vi "探头测量值显示.vi"(11 "校准参数":u16(ring) caption="校准参数：" items=["pH", "DO", "浊度", "电导率", "叶绿素a", "藻密度", "ORP", "COD", "DO2", "氯化物", "氨氮", "水中油", "悬浮物"]) -> (0 "线性系数":cluster{bool, "K":sgl, "B":sgl}, 1 "信号值":sgl, 2 "检测值":sgl, 3 "序列号":string, 4 "检测值.格式字符串":string, 5 "温度补偿系数":cluster{bool, "温度补偿系数":sgl}, 6 "信号值.格式字符串":string, 7 "电极状态标志":u16)   [LabVIEW 2022 SP3, in "斯坦道多参数.lvlib"]
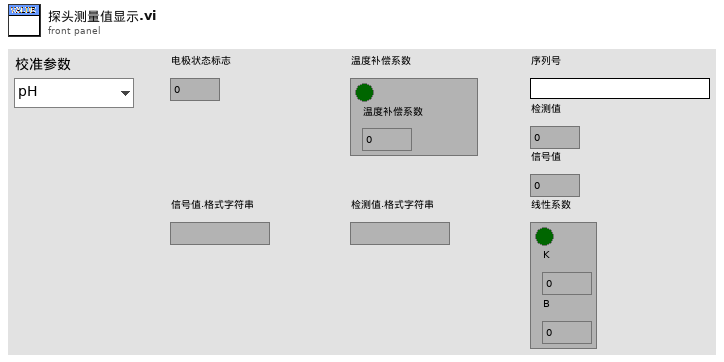
[diagram p1: front panel]
types:
  T1 = typedef "斯坦道多参数.lvlib/探头类型.ctl" = enum16{"禹山", "国弘", "纳清", "STD"}
  T2 = cluster{"pH探头选择":T1, "DO探头选择":T1, "电导率探头选择":T1, "浊度探头选择":T1, "悬浮物探头选择":T1, "叶绿素a探头选择":T1, "蓝绿藻探头选择":T1, "orp探头选择":T1, "COD探头选择":T1, "DO2探头选择":T1, "氨氮探头选择":T1, "水中油探头选择":T1, "余氯探头选择":T1}
  T3 = enum16{"null", "pH", "DO", "浊度", "电导率", "叶绿素a", "DO2"}
  T4 = enum16{"null", "pH", "DO", "浊度", "电导率", "叶绿素a", "DO2", "藻密度", "悬浮物"}
  T5 = enum16{"null", "pH", "DO", "浊度", "电导率", "叶绿素a", "DO2", "藻密度"}
  T6 = cluster{"输出值":cluster{"K":sgl, "B":sgl}, "SN":string}
  T7 = cluster{"电极状态标志":u16, "电极型号标志":u16, "酸碱度测量值":sgl, "温度测量值":sgl, "酸碱度信号值":sgl, "温度信号值":sgl, "酸碱度偏移修正值":sgl, "温度偏移修正值":sgl, "手动温度补偿值":sgl, "酸碱度电极零点":sgl, "酸碱度电极斜率":sgl, "第1点标准值记录":sgl, "第1点信号值记录":sgl, "第1点温度值记录":sgl, "第2点标准值记录":sgl, "第2点信号值记录":sgl, "第2点温度值记录":sgl, "命令滤波设定":u16, "温度模式":enum16{"ATC", "MTC"}, "生产批次":u16, "电极序号":u16, "串口地址":u16, "串口波特率":enum16{"9600", "19200", "115200"}, "串口校验位":enum16{"NONE", "ODD", "EVEN"}, "串口停止位":enum16{"1bit", "2bit"}, "第一点标准值":sgl, "第二点标准值":sgl}
  T8 = cluster{"报警码":u16, "pH数值":sgl, "0X0003_NC":sgl, "温度数据":sgl, "pH原始信号 mv":sgl, "0X0009_NC":string, "产品名称":string, "序列号":string, "硬件版本":string, "软件版本":string, "通讯地址":u16, "波特率":u16, "设备类型":u16, "0X0026_NC":string, "第一点原始数据":sgl, "第一点校准数据":sgl, "第二点原始数据":sgl, "第二点校准数据":sgl, "探头校准命令":u16, "温度校准参数":sgl, "温度校准命令":u16}
  T9 = cluster{"电极状态标志":u16, "电极型号标志":u16, "溶解氧测量值":sgl, "温度测量值":sgl, "溶解氧饱和度值":sgl, "盐度补偿值":sgl, "大气压补偿值":sgl, "溶解氧偏移修正值":sgl, "温度偏移修正值":sgl, "手动温度补偿值":sgl, "溶解氧电极零点":sgl, "溶解氧电极斜率":sgl, "第1点标准值记录":sgl, "第1点信号值记录":sgl, "第1点温度值记录":sgl, "第2点标准值记录":sgl, "第2点信号值记录":sgl, "第2点温度值记录":sgl, "命令滤波设定":u16, "温度模式":enum16{"ATC", "MTC"}, "生产批次":u16, "电极序号":u16, "串口地址":u16, "串口波特率":enum16{"9600", "19200", "115200"}, "串口校验位":enum16{"NONE", "ODD", "EVEN"}, "串口停止位":enum16{"1bit", "2bit"}, "第一点标准值":sgl, "第二点标准值":sgl}
  T10 = cluster{"报警码":u16, "溶解氧数值（mg/L）":sgl, "溶解氧数据（%）":sgl, "温度数据":sgl, "溶解氧原始信号 nA":sgl, "大气压力":sgl, "盐度":sgl, "0X0009_NC":string, "产品名称":string, "序列号":string, "硬件版本":string, "软件版本":string, "通讯地址":u16, "波特率":u16, "设备类型":u16, "0X0026_NC":string, "第一点原始数据":sgl, "第一点校准数据":sgl, "第二点原始数据":sgl, "第二点校准数据":sgl, "探头校准命令":u16, "温度校准参数":sgl, "温度校准命令":u16}
  T11 = cluster{"电极状态标志":u16, "电极型号标志":u16, "浊度测量值":sgl, "温度测量值":sgl, "浊度信号值":sgl, "浊度偏移修正值":sgl, "温度偏移修正值":sgl, "手动温度补偿值":sgl, "浊度电极零点":sgl, "浊度电极斜率":sgl, "清洁周期":u16, "命令滤波设定":u16, "温度模式":enum16{"ATC", "MTC"}, "生产批次":u16, "电极序号":u16, "串口地址":u16, "串口波特率":enum16{"9600", "19200", "115200"}, "串口校验位":enum16{"NONE", "ODD", "EVEN"}, "串口停止位":enum16{"1bit", "2bit"}, "第一点标准值":sgl, "第二点标准值":sgl, "第三点标准值":sgl}
  T12 = cluster{"报警码":u16, "浊度数值 NTU":sgl, "温度数据":sgl, "原始光强数值":u16, "量程":u16, "平均次数":u16, "清扫模式":u16, "清扫次数":u16, "清扫间隔分钟":u16, "0X000B_NC":string, "产品名称":string, "序列号":string, "硬件版本":string, "软件版本":string, "通讯地址":u16, "波特率":u16, "设备类型":u16, "0X0026_NC":string, "校准量程":u16, "第一点原始光强":u16, "第一点校准数据":sgl, "第二点原始光强":u16, "第二点校准数据":sgl, "第三点原始光强":u16, "第三点校准数据":sgl, "探头校准命令":u16, "温度校准参数":sgl, "温度校准命令":u16}
  T13 = cluster{"电极状态标志":u16, "电极型号标志":u16, "电导率测量值":sgl, "温度测量值":sgl, "电导率信号值":sgl, "温度信号值":sgl, "温度补偿系数":sgl, "电导率偏移修正值":sgl, "温度偏移修正值":sgl, "手动温度补偿值":sgl, "电导率电极零点":sgl, "电导率电极斜率":sgl, "命令滤波设定":u16, "温度模式":enum16{"ATC", "MTC"}, "生产批次":u16, "电极序号":u16, "串口地址":u16, "串口波特率":enum16{"9600", "19200", "115200"}, "串口校验位":enum16{"NONE", "ODD", "EVEN"}, "串口停止位":enum16{"1bit", "2bit"}, "第一点标准值":sgl, "第二点标准值":sgl}
  T14 = cluster{"报警码":u16, "电导率数据（uS/cm）":sgl, "0x0003 NC":sgl, "温度数据":sgl, "电导率原始信号电阻":sgl, "当前量程":u16, "温度补偿系数":sgl, "0X0009_NC":string, "产品名称":string, "序列号":string, "硬件版本":string, "软件版本":string, "通讯地址":u16, "波特率":u16, "设备类型":u16, "0X0026_NC":string, "第一点原始数据":sgl, "第一点校准数据":sgl, "0X0035_NC":sgl, "0X0037_NC":sgl, "探头校准命令":u16, "温度校准参数":sgl, "温度校准命令":u16}
  T15 = cluster{"报警码":u16, "叶绿素a":sgl, "温度数据":sgl, "原始光强数值":u16, "量程":u16, "平均次数":u16, "清扫模式":u16, "清扫次数":u16, "清扫间隔分钟":u16, "0X000B_NC":string, "产品名称":string, "序列号":string, "硬件版本":string, "软件版本":string, "通讯地址":u16, "波特率":u16, "设备类型":u16, "0X0026_NC":string, "校准量程":u16, "第一点原始光强":u16, "第一点校准数据":sgl, "第二点原始光强":u16, "第二点校准数据":sgl, "第三点原始光强":u16, "第三点校准数据":sgl, "探头校准命令":u16, "温度校准参数":sgl, "温度校准命令":u16}
  T16 = cluster{"报警码":u16, "蓝绿藻":sgl, "温度数据":sgl, "原始光强数值":u16, "量程":u16, "平均次数":u16, "清扫模式":u16, "清扫次数":u16, "清扫间隔分钟":u16, "0X000B_NC":string, "产品名称":string, "序列号":string, "硬件版本":string, "软件版本":string, "通讯地址":u16, "波特率":u16, "设备类型":u16, "0X0026_NC":string, "校准量程":u16, "第一点原始光强":u16, "第一点校准数据":sgl, "第二点原始光强":u16, "第二点校准数据":sgl, "第三点原始光强":u16, "第三点校准数据":sgl, "探头校准命令":u16, "温度校准参数":sgl, "温度校准命令":u16}
  T17 = cluster{"电极状态标志":u16, "电极型号标志":u16, "测量值":sgl, "温度测量值":sgl, "信号值":sgl, "温度信号值":sgl, "000AH_NC":sgl, "偏移修正值":sgl, "温度偏移修正值":sgl, "手动温度补偿值":sgl, "命令滤波设定":u16, "温度模式":enum16{"ATC", "MTC"}, "生产批次":u16, "传感器序号":u16, "串口地址":u16, "串口波特率":enum16{"9600", "19200", "115200"}, "串口校验位":enum16{"NONE", "ODD", "EVEN"}, "串口停止位":enum16{"1bit", "2bit"}}
  T18 = cluster{"电极状态标志":u16, "电极型号标志":u16, "COD测量值":sgl, "浊度测量值":sgl, "COD信号值":sgl, "浊度信号值":sgl, "温度测量值":sgl, "COD偏移修正值":sgl, "浊度偏移修正值":sgl, "COD水样校正值":sgl, "温度偏移修正值":sgl, "COD零点系数":sgl, "COD斜率系数":sgl, "浊度零点系数":sgl, "浊度斜率系数":sgl, "COD测值K值":sgl, "浊度测值K值":sgl, "浊度补偿COD系数值":sgl, "COD温度补偿系数值 ":sgl, "测量周期":u16, "清洗周期":u16, "命令寄存器":u16, "数字滤波设定":u16, "温度模式":enum16{"AUTO", "OFF"}, "生产批次":u16, "电极序号":u16, "串口地址":u16, "串口波特率":enum16{"9600", "19200", "115200"}, "串口校验位":enum16{"NONE", "ODD", "EVEN"}, "串口停止位":enum16{"1bit", "2bit"}, "第一点校正指令":u16, "第一点标准值":sgl, "第二点校正指令":u16, "第二点标准值":sgl, "第三点校正指令":u16, "第三点标准值":sgl, "COD吸光度":sgl, "浊度吸光度":sgl, "温度信号值":sgl}
  T19 = cluster{"电极状态标志":u16, "电极型号标志":u16, "测量值":sgl, "温度测量值":sgl, "信号值":sgl, "温度信号值":sgl, "偏移修正值":sgl, "温度偏移修正值":sgl, "手动温度补偿值":sgl, "电极零点":sgl, "电极斜率":sgl, "第1点标准值记录":sgl, "第1点信号值记录":sgl, "第1点温度值记录":sgl, "第2点标准值记录":sgl, "第2点信号值记录":sgl, "第2点温度值记录":sgl, "命令滤波设定":u16, "温度模式":enum16{"ATC", "MTC"}, "生产批次":u16, "电极序号":u16, "串口地址":u16, "串口波特率":enum16{"9600", "19200", "115200"}, "串口校验位":enum16{"NONE", "ODD", "EVEN"}, "串口停止位":enum16{"1bit", "2bit"}, "第一点标准值":sgl, "第二点标准值":sgl}
  T20 = cluster{"报警码":u16, "参数1数据":sgl, "参数2数据":sgl, "参数3数据":sgl, "参数4数据":sgl, "温度数据":sgl, "参数1原始信号":sgl, "参数2原始信号":sgl, "参数3原始信号":sgl, "参数4原始信号":sgl, "序列号":string, "硬件版本":string, "软件版本":string, "通讯地址":u16, "波特率":u16, "设备类型":u16, "0X0026_NC":string, "校准参数类型":u16, "第一点原始数据":sgl, "第一点校准数据":sgl, "第二点原始数据":sgl, "第二点校准数据":sgl, "探头校准命令":u16, "温度校准参数":sgl, "温度校准命令":u16}
  T21 = cluster{"电极状态标志":u16, "电极型号标志":u16, "测量值":sgl, "温度测量值":sgl, "信号值":sgl, "水中油B值":sgl, "温度B值":sgl, "水中油零点系数":sgl, "水中油斜率系数":sgl, "水中油K值":sgl, "空白电位值":sgl, "温度信号值":sgl, "温度补偿系数":sgl, "测量档位":u16, "清洁周期":u16, "命令寄存器":u16, "数位滤波设定":u16, "温度模式":enum16{"ATC", "MTC"}, "生产批次":u16, "电极序号":u16, "串口地址":u16, "串口波特率":enum16{"9600", "19200", "115200"}, "串口校验位":enum16{"NONE", "ODD", "EVEN"}, "串口停止位":enum16{"1bit", "2bit"}, "第一点校正指令":u16, "第一点标准值":sgl, "第二点校正指令":u16, "第二点标准值":sgl, "第三点校正指令":u16, "第三点标准值":sgl}
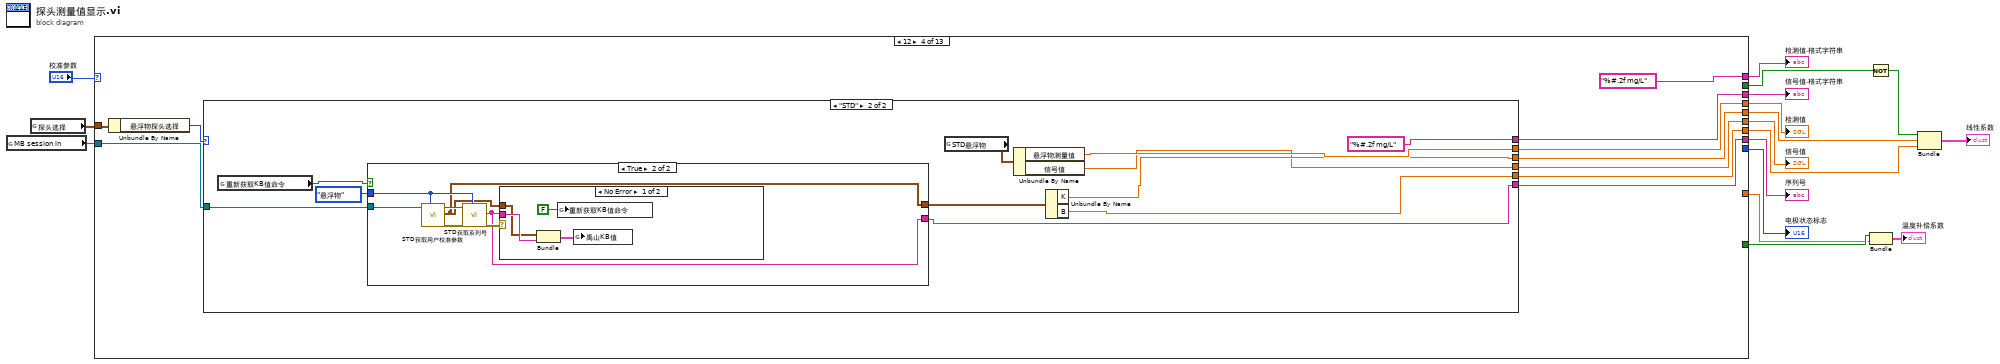
[diagram p0: block diagram]
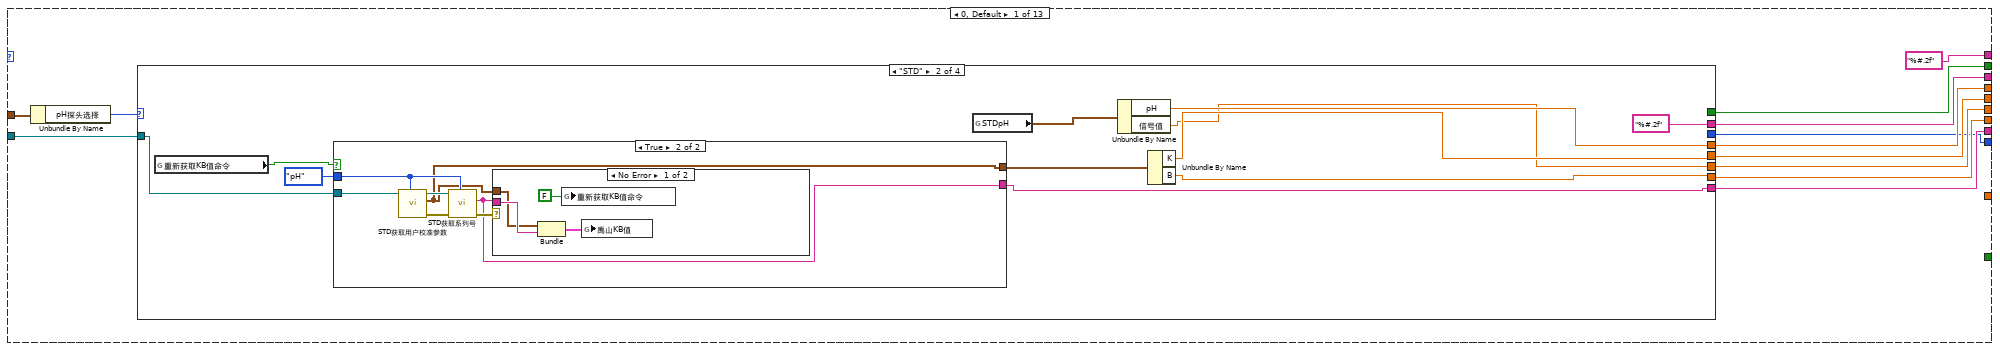
[diagram p2: hidden frame]
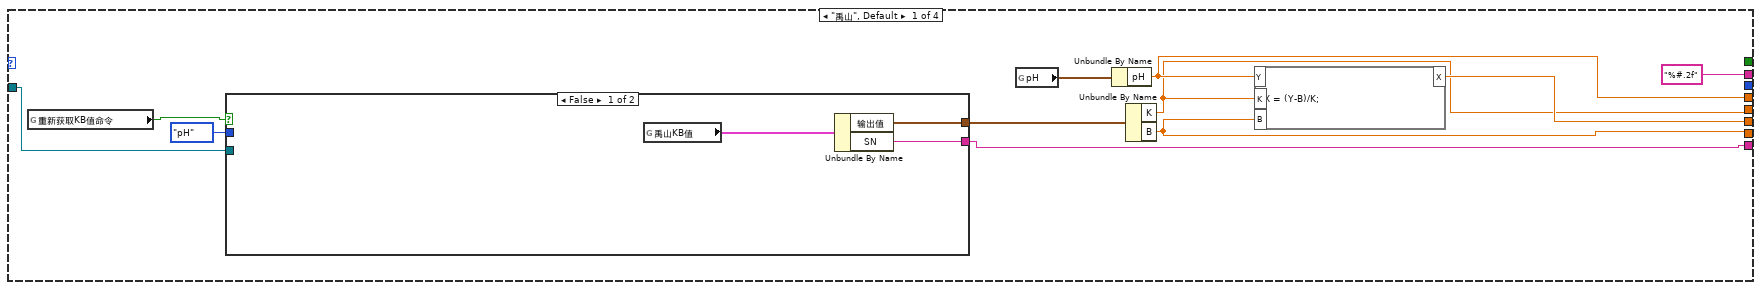
[diagram p3: hidden frame]
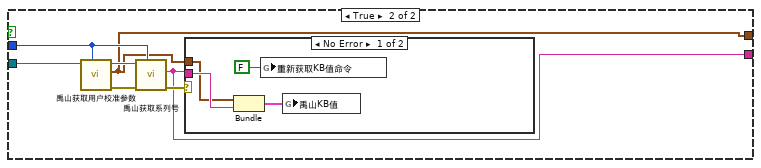
[diagram p4: hidden frame]
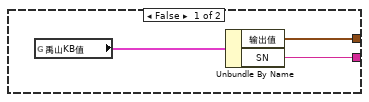
[diagram p6: hidden frame]
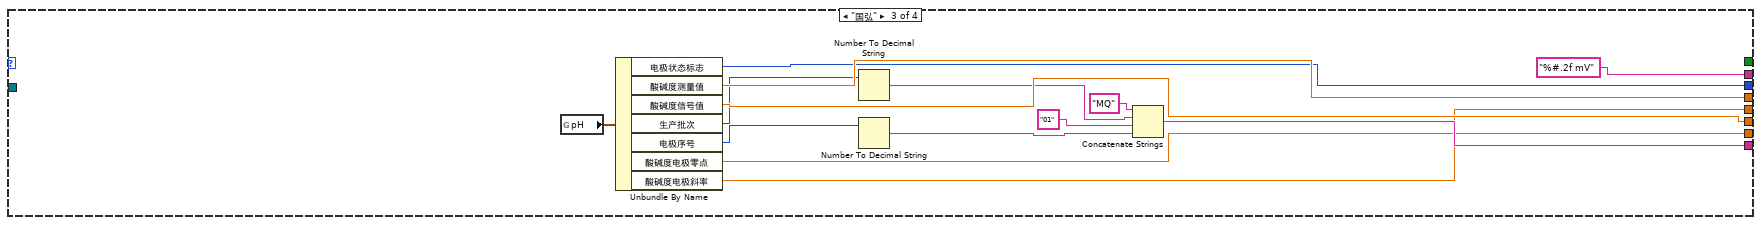
[diagram p8: hidden frame]
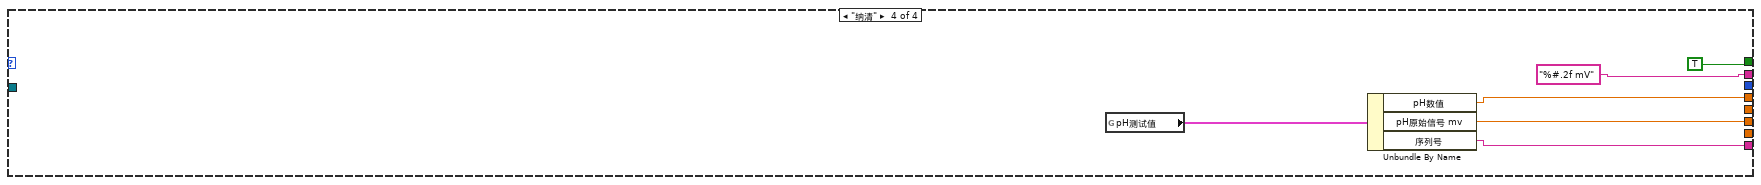
[diagram p9: hidden frame]
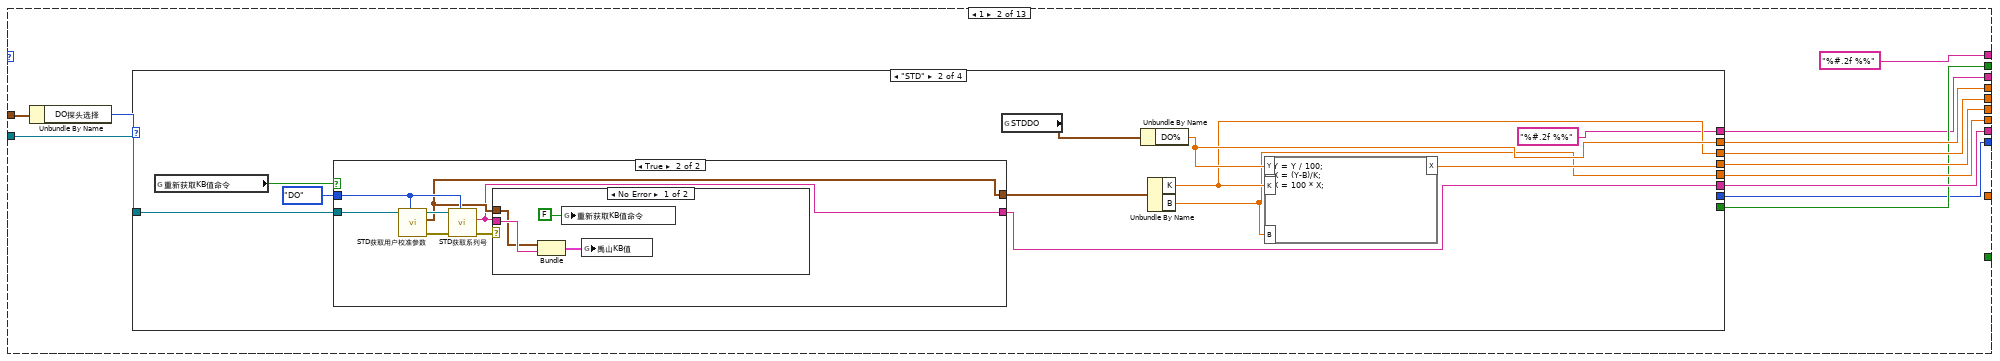
[diagram p10: hidden frame]
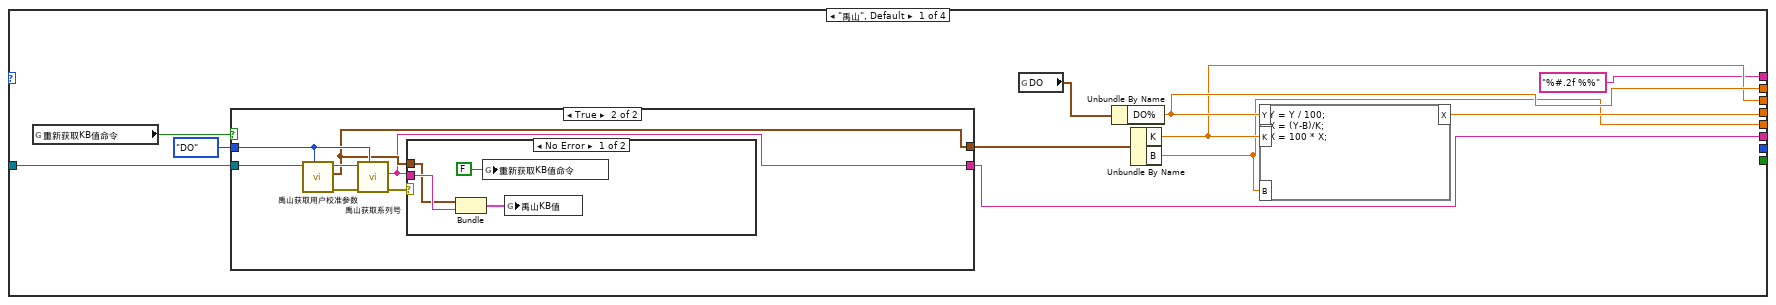
[diagram p11: hidden frame]
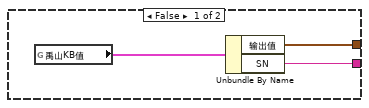
[diagram p12: hidden frame]
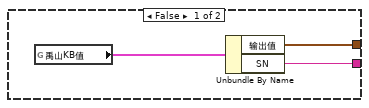
[diagram p14: hidden frame]
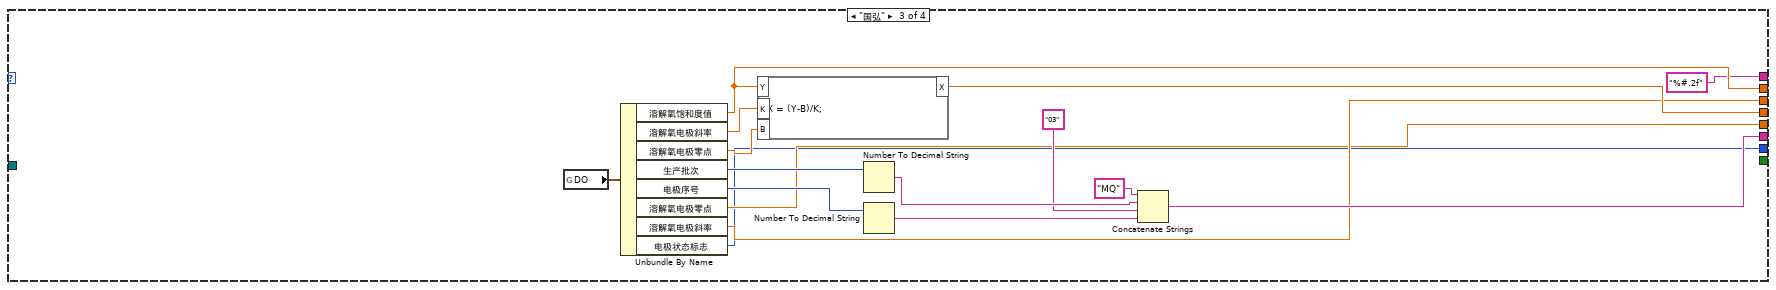
[diagram p16: hidden frame]
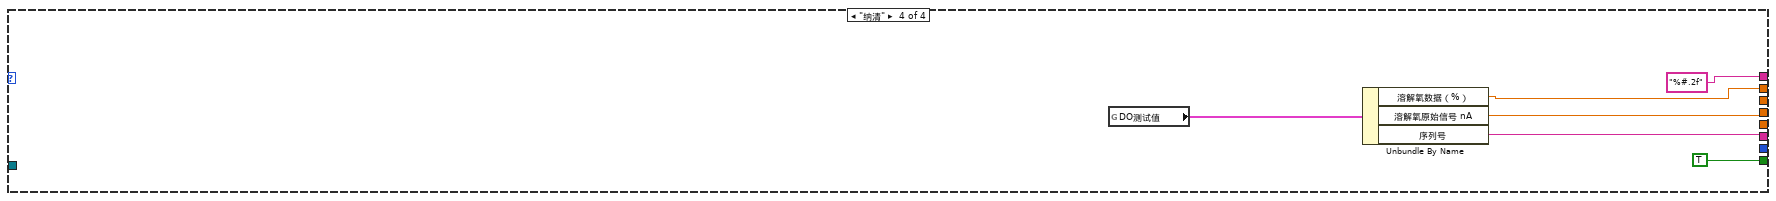
[diagram p17: hidden frame]
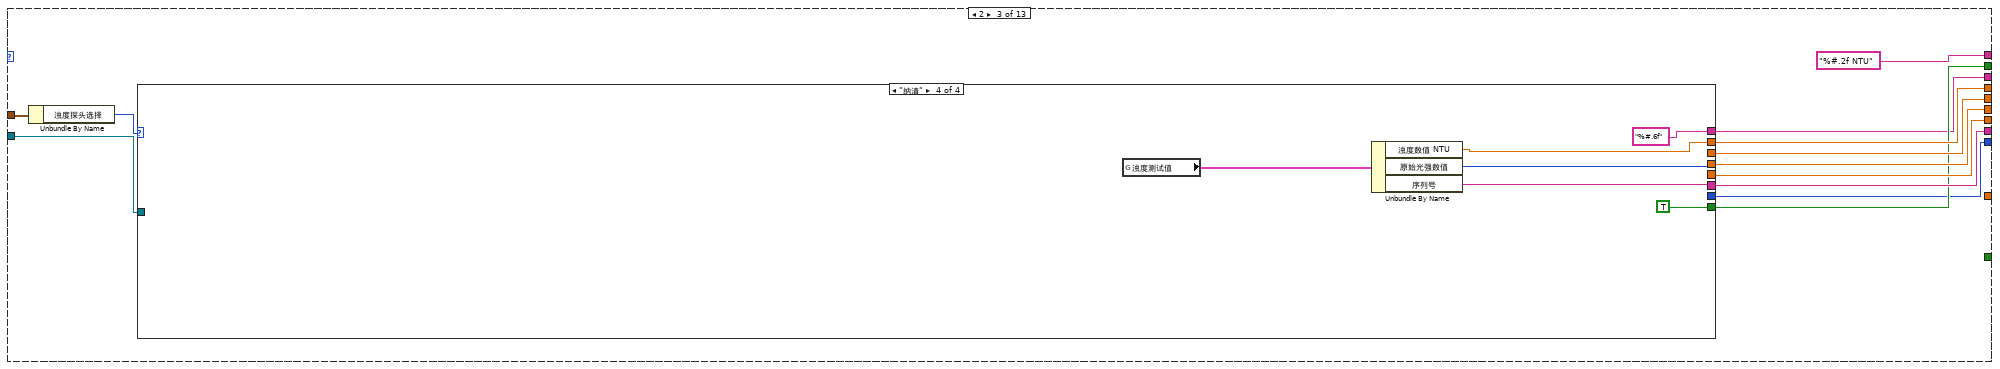
[diagram p18: hidden frame]
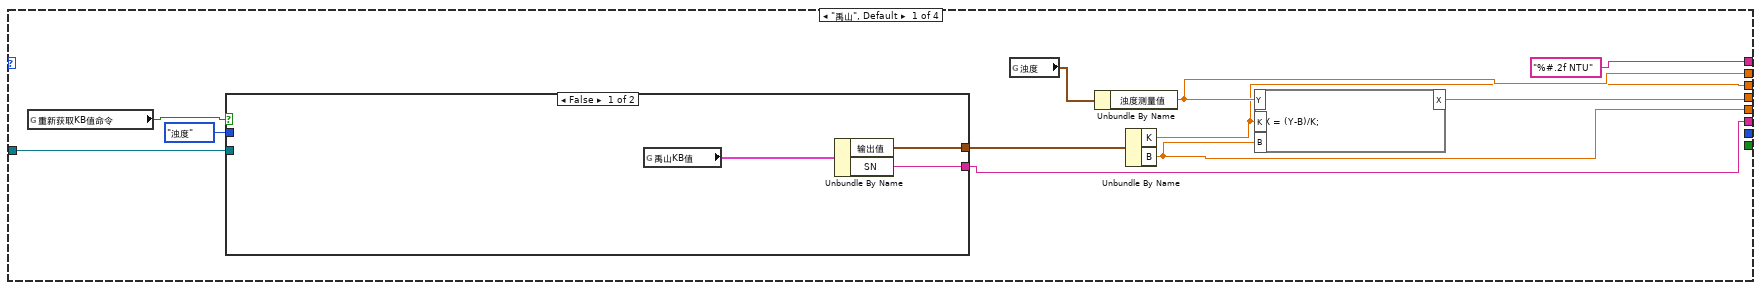
[diagram p19: hidden frame]
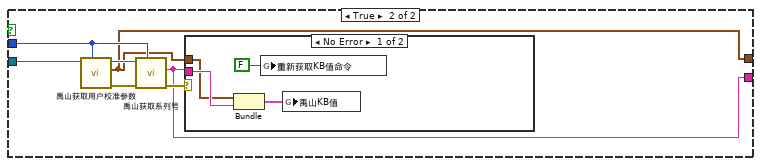
[diagram p20: hidden frame]
diagram:
  n1 = global read "多参数全局变量.vi" "MB session in"() -> (w13:refnum<class "MB_Master.lvclass">)
  n2 = global read "断电保存变量.vi" "探头选择"() -> (w15:T2)
  n3 = case shown="12" "校准参数" {
    tunnel: [w28 w110 w194 w274 w313 w398 w469 w520 w554 w565 w596 w603 w618] -> w17
    tunnel: w15 -> [w27 w109 w193 w273 w312 w397 w468 w519 _ _ _ _ _]
    tunnel: [w26 w108 w192 w272 w311 w396 w467 w518 w553 w566 w595 w602 w617] -> w14
    tunnel: w13 -> [w25 w107 w191 w271 w310 w395 w462 _ _ w563 _ _ _]
    tunnel: [w24 w106 w190 w270 w309 w394 w466 w517 w552 w564 w594 w601 w616] -> w12
    tunnel: [w23 w105 w189 w269 w308 w393 w461 sgl 0.0 ("K") w551 w559 w593 _ w615] -> w9
    tunnel: [w22 w104 w188 w268 w307 w392 w460 sgl 0.0 ("B") w550 w558 w592 _ w614] -> w8
    tunnel: [w21 w103 w187 _ w306 w391 w465 w516 _ FALSE _ TRUE _] -> w11
    tunnel: ["%#.2f" ("数值文本.格式字符串") "%#.2f %%" ("数值文本.格式字符串") "%#.2f NTU" ("数值文本.格式字符串") "%#.2f mg/L" ("数值文本.格式字符串") "%#.2f μS/cm" ("数值文本.格式字符串") "%#.2f μg/L" ("数值文本.格式字符串") "%#.2f cells/mL" ("数值文本.格式字符串") "%#.2f mV" ("数值文本.格式字符串") "%#.2f" ("数值文本.格式字符串") "%#.2f %%" ("数值文本.格式字符串") "%#.2f" ("数值文本.格式字符串") "%#.2f" ("数值文本.格式字符串") "%#.2f" ("数值文本.格式字符串")] -> w6
    tunnel: [_ _ _ _ w304 _ _ _ _ _ _ _ _] -> w4
    tunnel: [_ _ _ _ w303 _ _ _ _ _ _ _ _] -> w5
    tunnel: [w19 w101 w185 _ w302 _ _ w512 w548 _ w590 _ w612] -> w2
    tunnel: [w18 w100 w184 w266 w301 w389 w463 "%#.2f mV" ("数值文本.格式字符串") "%#.2f mV" ("数值文本.格式字符串") "%#.2f %%" ("数值文本.格式字符串") "%#.2f mV" ("数值文本.格式字符串") "%#.2f mV" ("数值文本.格式字符串") "%#.2f mV" ("数值文本.格式字符串")] -> w1
    frame 0, Default {
      n4 = Unbundle By Name(w27) -> ("pH探头选择"=w29:T1)
      n5 = case shown="\"STD\"" w29 {
        tunnel: [w39 w64 w92 w99] -> w28
        tunnel: [w38 w55 w91 w97] -> w26
        tunnel: w25 -> [w36 w62 _ _]
        tunnel: [w37 w63 w84 w96] -> w24
        tunnel: [w33 w59 w83 _] -> w23
        tunnel: [w32 w58 w82 _] -> w22
        tunnel: [_ _ _ TRUE] -> w21
        tunnel: [_ _ w81 _] -> w19
        tunnel: ["%#.2f" ("数值文本.格式字符串") "%#.2f" ("数值文本.格式字符串") "%#.2f mV" ("数值文本.格式字符串") "%#.2f mV" ("数值文本.格式字符串")] -> w18
        frame "禹山", Default {
          n6 = global read "多参数全局变量.vi" "重新获取KB值命令"() -> (w30:bool)
          n7 = case shown="False" w30 {
            tunnel: [w41 w45] -> w37
            tunnel: w36 -> [_ w50]
            tunnel: T3."pH" ("探头") -> [_ w49]
            tunnel: [w42 w44] -> w34
            frame False {
              n8 = global read "多参数全局变量.vi" "禹山KB值"() -> (w43:T6)
              n9 = Unbundle By Name(w43) -> ("输出值"=w42:cluster{"K":sgl, "B":sgl}, "SN"=w41:string)
            }
            frame True {
              n10 = call "禹山获取用户校准参数.vi"("探头"=w49, "MB session in"=w50) -> ("error out"=w47:errorcluster, "输出值"=w44:cluster{"K":sgl, "B":sgl}, "MB session out"=w48:refnum<class "MB_Master.lvclass">)  [unwired: 7 in]
              n11 = call "禹山获取系列号.vi"("探头"=w49, "error in (no error)"=w47, "MB session in"=w48) -> ("error out"=w46:errorcluster, "SN"=w45:string)  [unwired: 6 in, 1 out]
              n12 = case shown="No Error" w46 {
                tunnel: w44 -> [w53 _]
                tunnel: w45 -> [w54 _]
                frame No Error {
                  n13 = Bundle("输出值"=w53, "SN"=w54) -> (w52:T6)  [unwired: 1 in]
                  n14 = global write "多参数全局变量.vi" "重新获取KB值命令"(FALSE ("重新获取KB值命令")) -> ()
                  n15 = global write "多参数全局变量.vi" "禹山KB值"(w52) -> ()
                }
                frame Error {
                }
              }
            }
          }
          n16 = global read "禹山过程全局变量.vi" "pH"() -> (w40:cluster{"温度测量值":sgl, "ORP":sgl, "pH":sgl})
          n17 = Unbundle By Name(w40) -> ("pH"=w39:sgl)
          n18 = Unbundle By Name(w34) -> ("K"=w33:sgl, "B"=w32:sgl)
          n19 = formula code="X = (Y-B)/K;"("Y"=w39, "K"=w33, "B"=w32) -> ("X"=w38:dbl)
        }
        frame "STD" {
          n20 = global read "多参数全局变量.vi" "重新获取KB值命令"() -> (w56:bool)
          n21 = case shown="True" w56 {
            tunnel: [w66 w70] -> w63
            tunnel: w62 -> [_ w75]
            tunnel: T3."pH" ("探头") -> [_ w74]
            tunnel: [w67 w69] -> w60
            frame False {
              n22 = global read "多参数全局变量.vi" "禹山KB值"() -> (w68:T6)
              n23 = Unbundle By Name(w68) -> ("输出值"=w67:cluster{"K":sgl, "B":sgl}, "SN"=w66:string)
            }
            frame True {
              n24 = call "STD获取用户校准参数.vi"("探头"=w74, "MB session in"=w75) -> ("error out"=w72:errorcluster, "输出值"=w69:cluster{"K":sgl, "B":sgl}, "MB session out"=w73:refnum<class "MB_Master.lvclass">)  [unwired: 7 in]
              n25 = call "STD获取系列号.vi"("探头"=w74, "error in (no error)"=w72, "MB session in"=w73) -> ("error out"=w71:errorcluster, "SN"=w70:string)  [unwired: 6 in, 1 out]
              n26 = case shown="No Error" w71 {
                tunnel: w69 -> [w78 _]
                tunnel: w70 -> [w79 _]
                frame No Error {
                  n27 = Bundle("输出值"=w78, "SN"=w79) -> (w77:T6)  [unwired: 1 in]
                  n28 = global write "多参数全局变量.vi" "重新获取KB值命令"(FALSE ("重新获取KB值命令")) -> ()
                  n29 = global write "多参数全局变量.vi" "禹山KB值"(w77) -> ()
                }
                frame Error {
                }
              }
            }
          }
          n30 = global read "禹山过程全局变量.vi" "STDpH"() -> (w65:cluster{"温度测量值":sgl, "pH":sgl, "信号值":sgl})
          n31 = Unbundle By Name(w65) -> ("pH"=w64:sgl, "信号值"=w55:sgl)
          n32 = Unbundle By Name(w60) -> ("K"=w59:sgl, "B"=w58:sgl)
        }
        frame "国弘" {
          n33 = global read "国弘过程全局变量.vi" "pH"() -> (w93:T7)
          n34 = Unbundle By Name(w93) -> ("电极状态标志"=w81:u16, "酸碱度测量值"=w92:sgl, "酸碱度信号值"=w91:sgl, "生产批次"=w86:u16, "电极序号"=w85:u16, "酸碱度电极零点"=w82:sgl, "酸碱度电极斜率"=w83:sgl)
          n35 = Number To Decimal String(number=w86) -> (decimal integer string=w90:string)  [unwired: 1 in]
          n36 = Number To Decimal String(number=w85) -> (decimal integer string=w88:string)  [unwired: 1 in]
          n37 = Concatenate Strings("MQ" ("字符串"), w90, "01" ("字符串"), w88) -> (w84:string)
        }
        frame "纳清" {
          n38 = global read "纳清过程全局变量.vi" "pH测试值"() -> (w98:T8)
          n39 = Unbundle By Name(w98) -> ("pH数值"=w99:sgl, "pH原始信号 mv"=w97:sgl, "序列号"=w96:string)
        }
      }
    }
    frame 1 {
      n40 = Unbundle By Name(w109) -> ("DO探头选择"=w111:T1)
      n41 = case shown="\"STD\"" w111 {
        tunnel: [w121 w146 w175 w183] -> w110
        tunnel: [w120 w145 w173 w181] -> w108
        tunnel: w107 -> [w118 w143 _ _]
        tunnel: [w119 w144 w166 w180] -> w106
        tunnel: [w115 w140 w165 _] -> w105
        tunnel: [w114 w139 w164 _] -> w104
        tunnel: [_ _ _ TRUE] -> w103
        tunnel: [_ _ w163 _] -> w101
        tunnel: ["%#.2f %%" ("数值文本.格式字符串") "%#.2f %%" ("数值文本.格式字符串") "%#.2f" ("数值文本.格式字符串") "%#.2f" ("数值文本.格式字符串")] -> w100
        frame "禹山", Default {
          n42 = global read "多参数全局变量.vi" "重新获取KB值命令"() -> (w112:bool)
          n43 = case shown="True" w112 {
            tunnel: [w123 w126] -> w119
            tunnel: w118 -> [_ w132]
            tunnel: [w124 w127] -> w117
            tunnel: T3."DO" ("探头") -> [_ w129]
            frame False {
              n44 = global read "多参数全局变量.vi" "禹山KB值"() -> (w125:T6)
              n45 = Unbundle By Name(w125) -> ("输出值"=w124:cluster{"K":sgl, "B":sgl}, "SN"=w123:string)
            }
            frame True {
              n46 = call "禹山获取用户校准参数.vi"("探头"=w129, "MB session in"=w132) -> ("error out"=w131:errorcluster, "输出值"=w127:cluster{"K":sgl, "B":sgl}, "MB session out"=w130:refnum<class "MB_Master.lvclass">)  [unwired: 7 in]
              n47 = call "禹山获取系列号.vi"("探头"=w129, "error in (no error)"=w131, "MB session in"=w130) -> ("error out"=w128:errorcluster, "SN"=w126:string)  [unwired: 6 in, 1 out]
              n48 = case shown="No Error" w128 {
                tunnel: w127 -> [w135 _]
                tunnel: w126 -> [w136 _]
                frame No Error {
                  n49 = Bundle("输出值"=w135, "SN"=w136) -> (w134:T6)  [unwired: 1 in]
                  n50 = global write "多参数全局变量.vi" "重新获取KB值命令"(FALSE ("重新获取KB值命令")) -> ()
                  n51 = global write "多参数全局变量.vi" "禹山KB值"(w134) -> ()
                }
                frame Error {
                }
              }
            }
          }
          n52 = global read "禹山过程全局变量.vi" "DO"() -> (w122:cluster{"温度测量值":sgl, "DO%":sgl, "DOmg/L":sgl})
          n53 = Unbundle By Name(w122) -> ("DO%"=w121:sgl)
          n54 = Unbundle By Name(w117) -> ("K"=w115:sgl, "B"=w114:sgl)
          n55 = formula code="Y = Y / 100;\nX = (Y-B)/K;\nX = 100 * X;"("Y"=w121, "K"=w115, "B"=w114) -> ("X"=w120:dbl)
        }
        frame "STD" {
          n56 = global read "多参数全局变量.vi" "重新获取KB值命令"() -> (w137:bool)
          n57 = case shown="True" w137 {
            tunnel: [w148 w151] -> w144
            tunnel: w143 -> [_ w157]
            tunnel: [w149 w152] -> w142
            tunnel: T3."DO" ("探头") -> [_ w154]
            frame False {
              n58 = global read "多参数全局变量.vi" "禹山KB值"() -> (w150:T6)
              n59 = Unbundle By Name(w150) -> ("输出值"=w149:cluster{"K":sgl, "B":sgl}, "SN"=w148:string)
            }
            frame True {
              n60 = call "STD获取用户校准参数.vi"("探头"=w154, "MB session in"=w157) -> ("error out"=w156:errorcluster, "输出值"=w152:cluster{"K":sgl, "B":sgl}, "MB session out"=w155:refnum<class "MB_Master.lvclass">)  [unwired: 7 in]
              n61 = call "STD获取系列号.vi"("探头"=w154, "error in (no error)"=w156, "MB session in"=w155) -> ("error out"=w153:errorcluster, "SN"=w151:string)  [unwired: 6 in, 1 out]
              n62 = case shown="No Error" w153 {
                tunnel: w152 -> [w160 _]
                tunnel: w151 -> [w161 _]
                frame No Error {
                  n63 = Bundle("输出值"=w160, "SN"=w161) -> (w159:T6)  [unwired: 1 in]
                  n64 = global write "多参数全局变量.vi" "重新获取KB值命令"(FALSE ("重新获取KB值命令")) -> ()
                  n65 = global write "多参数全局变量.vi" "禹山KB值"(w159) -> ()
                }
                frame Error {
                }
              }
            }
          }
          n66 = global read "禹山过程全局变量.vi" "STDDO"() -> (w147:cluster{"温度测量值":sgl, "DO%":sgl, "DOmg/L":sgl})
          n67 = Unbundle By Name(w147) -> ("DO%"=w146:sgl)
          n68 = Unbundle By Name(w142) -> ("K"=w140:sgl, "B"=w139:sgl)
          n69 = formula code="Y = Y / 100;\nX = (Y-B)/K;\nX = 100 * X;"("Y"=w146, "K"=w140, "B"=w139) -> ("X"=w145:dbl)
        }
        frame "国弘" {
          n70 = global read "国弘过程全局变量.vi" "DO"() -> (w177:T9)
          n71 = Unbundle By Name(w177) -> ("溶解氧饱和度值"=w175:sgl, "溶解氧电极斜率"=w176:sgl, "溶解氧电极零点"=w174:sgl, "生产批次"=w167:u16, "电极序号"=w168:u16, "溶解氧电极零点"=w164:sgl, "溶解氧电极斜率"=w165:sgl, "电极状态标志"=w163:u16)
          n72 = formula code="X = (Y-B)/K;"("Y"=w175, "K"=w176, "B"=w174) -> ("X"=w173:dbl)
          n73 = Number To Decimal String(number=w167) -> (decimal integer string=w172:string)  [unwired: 1 in]
          n74 = Number To Decimal String(number=w168) -> (decimal integer string=w170:string)  [unwired: 1 in]
          n75 = Concatenate Strings("MQ" ("字符串"), w172, "03" ("字符串"), w170) -> (w166:string)
        }
        frame "纳清" {
          n76 = global read "纳清过程全局变量.vi" "DO测试值"() -> (w182:T10)
          n77 = Unbundle By Name(w182) -> ("溶解氧数据（%）"=w183:sgl, "溶解氧原始信号 nA"=w181:sgl, "序列号"=w180:string)
        }
      }
    }
    frame 2 {
      n78 = Unbundle By Name(w193) -> ("浊度探头选择"=w195:T1)
      n79 = case shown="\"纳清\"" w195 {
        tunnel: [w205 w230 w258 w265] -> w194
        tunnel: [w204 w221 w257 w263] -> w192
        tunnel: w191 -> [w202 w228 _ _]
        tunnel: [w203 w229 w252 w262] -> w190
        tunnel: [w199 w225 w249 _] -> w189
        tunnel: [w198 w224 w248 _] -> w188
        tunnel: [_ _ _ TRUE] -> w187
        tunnel: [_ _ w247 _] -> w185
        tunnel: ["%#.2f NTU" ("数值文本.格式字符串") "%#.2f NTU" ("数值文本.格式字符串") "%#.2f NTU" ("数值文本.格式字符串") "%#.6f" ("数值文本.格式字符串")] -> w184
        frame "禹山", Default {
          n80 = global read "多参数全局变量.vi" "重新获取KB值命令"() -> (w196:bool)
          n81 = case shown="False" w196 {
            tunnel: [w207 w211] -> w203
            tunnel: w202 -> [_ w216]
            tunnel: [w208 w210] -> w201
            tunnel: T3."浊度" ("探头") -> [_ w213]
            frame False {
              n82 = global read "多参数全局变量.vi" "禹山KB值"() -> (w209:T6)
              n83 = Unbundle By Name(w209) -> ("输出值"=w208:cluster{"K":sgl, "B":sgl}, "SN"=w207:string)
            }
            frame True {
              n84 = call "禹山获取用户校准参数.vi"("探头"=w213, "MB session in"=w216) -> ("error out"=w214:errorcluster, "输出值"=w210:cluster{"K":sgl, "B":sgl}, "MB session out"=w215:refnum<class "MB_Master.lvclass">)  [unwired: 7 in]
              n85 = call "禹山获取系列号.vi"("探头"=w213, "error in (no error)"=w214, "MB session in"=w215) -> ("error out"=w212:errorcluster, "SN"=w211:string)  [unwired: 6 in, 1 out]
              n86 = case shown="No Error" w212 {
                tunnel: w210 -> [w219 _]
                tunnel: w211 -> [w220 _]
                frame No Error {
                  n87 = Bundle("输出值"=w219, "SN"=w220) -> (w218:T6)  [unwired: 1 in]
                  n88 = global write "多参数全局变量.vi" "重新获取KB值命令"(FALSE ("重新获取KB值命令")) -> ()
                  n89 = global write "多参数全局变量.vi" "禹山KB值"(w218) -> ()
                }
                frame Error {
                }
              }
            }
          }
          n90 = global read "禹山过程全局变量.vi" "浊度"() -> (w206:cluster{"温度测量值":sgl, "浊度测量值":sgl})
          n91 = Unbundle By Name(w206) -> ("浊度测量值"=w205:sgl)
          n92 = Unbundle By Name(w201) -> ("K"=w199:sgl, "B"=w198:sgl)
          n93 = formula code="X = (Y-B)/K;"("Y"=w205, "K"=w199, "B"=w198) -> ("X"=w204:dbl)
        }
        frame "STD" {
          n94 = global read "多参数全局变量.vi" "重新获取KB值命令"() -> (w222:bool)
          n95 = case shown="True" w222 {
            tunnel: [w232 w236] -> w229
            tunnel: w228 -> [_ w241]
            tunnel: [w233 w235] -> w227
            tunnel: T3."浊度" ("探头") -> [_ w238]
            frame False {
              n96 = global read "多参数全局变量.vi" "禹山KB值"() -> (w234:T6)
              n97 = Unbundle By Name(w234) -> ("输出值"=w233:cluster{"K":sgl, "B":sgl}, "SN"=w232:string)
            }
            frame True {
              n98 = call "STD获取用户校准参数.vi"("探头"=w238, "MB session in"=w241) -> ("error out"=w239:errorcluster, "输出值"=w235:cluster{"K":sgl, "B":sgl}, "MB session out"=w240:refnum<class "MB_Master.lvclass">)  [unwired: 7 in]
              n99 = call "STD获取系列号.vi"("探头"=w238, "error in (no error)"=w239, "MB session in"=w240) -> ("error out"=w237:errorcluster, "SN"=w236:string)  [unwired: 6 in, 1 out]
              n100 = case shown="No Error" w237 {
                tunnel: w235 -> [w244 _]
                tunnel: w236 -> [w245 _]
                frame No Error {
                  n101 = Bundle("输出值"=w244, "SN"=w245) -> (w243:T6)  [unwired: 1 in]
                  n102 = global write "多参数全局变量.vi" "重新获取KB值命令"(FALSE ("重新获取KB值命令")) -> ()
                  n103 = global write "多参数全局变量.vi" "禹山KB值"(w243) -> ()
                }
                frame Error {
                }
              }
            }
          }
          n104 = global read "禹山过程全局变量.vi" "STD浊度"() -> (w231:cluster{"温度测量值":sgl, "浊度测量值":sgl, "信号值":sgl})
          n105 = Unbundle By Name(w231) -> ("浊度测量值"=w230:sgl, "信号值"=w221:sgl)
          n106 = Unbundle By Name(w227) -> ("K"=w225:sgl, "B"=w224:sgl)
        }
        frame "国弘" {
          n107 = global read "国弘过程全局变量.vi" "Turb"() -> (w259:T11)
          n108 = Unbundle By Name(w259) -> ("浊度测量值"=w258:sgl, "浊度信号值"=w257:sgl, "生产批次"=w250:u16, "电极序号"=w251:u16, "浊度电极零点"=w248:sgl, "浊度电极斜率"=w249:sgl, "电极状态标志"=w247:u16)
          n109 = Number To Decimal String(number=w250) -> (decimal integer string=w256:string)  [unwired: 1 in]
          n110 = Number To Decimal String(number=w251) -> (decimal integer string=w254:string)  [unwired: 1 in]
          n111 = Concatenate Strings("MQ" ("字符串"), w256, "04" ("字符串"), w254) -> (w252:string)
        }
        frame "纳清" {
          n112 = global read "纳清过程全局变量.vi" "浊度测试值"() -> (w264:T12)
          n113 = Unbundle By Name(w264) -> ("浊度数值 NTU"=w265:sgl, "原始光强数值"=w263:u16, "序列号"=w262:string)
        }
      }
    }
    frame 12 {
      n114 = Unbundle By Name(w273) -> ("悬浮物探头选择"=w275:T1)
      n115 = case shown="\"STD\"" w275 {
        tunnel: [_ w285] -> w274
        tunnel: [_ w277] -> w272
        tunnel: w271 -> [_ w283]
        tunnel: [_ w284] -> w270
        tunnel: [_ w281] -> w269
        tunnel: [_ w280] -> w268
        tunnel: [_ "%#.2f mg/L" ("数值文本.格式字符串")] -> w266
        frame Default {
        }
        frame "STD" {
          n116 = global read "多参数全局变量.vi" "重新获取KB值命令"() -> (w278:bool)
          n117 = case shown="True" w278 {
            tunnel: [w287 w291] -> w284
            tunnel: w283 -> [_ w296]
            tunnel: [w288 w290] -> w282
            tunnel: T4."悬浮物" ("探头") -> [_ w293]
            frame False {
              n118 = global read "多参数全局变量.vi" "禹山KB值"() -> (w289:T6)
              n119 = Unbundle By Name(w289) -> ("输出值"=w288:cluster{"K":sgl, "B":sgl}, "SN"=w287:string)
            }
            frame True {
              n120 = call "STD获取用户校准参数.vi"("探头"=w293, "MB session in"=w296) -> ("error out"=w294:errorcluster, "输出值"=w290:cluster{"K":sgl, "B":sgl}, "MB session out"=w295:refnum<class "MB_Master.lvclass">)  [unwired: 7 in]
              n121 = call "STD获取系列号.vi"("探头"=w293, "error in (no error)"=w294, "MB session in"=w295) -> ("error out"=w292:errorcluster, "SN"=w291:string)  [unwired: 6 in, 1 out]
              n122 = case shown="No Error" w292 {
                tunnel: w290 -> [w299 _]
                tunnel: w291 -> [w300 _]
                frame No Error {
                  n123 = Bundle("输出值"=w299, "SN"=w300) -> (w298:T6)  [unwired: 1 in]
                  n124 = global write "多参数全局变量.vi" "重新获取KB值命令"(FALSE ("重新获取KB值命令")) -> ()
                  n125 = global write "多参数全局变量.vi" "禹山KB值"(w298) -> ()
                }
                frame Error {
                }
              }
            }
          }
          n126 = global read "禹山过程全局变量.vi" "STD悬浮物"() -> (w286:cluster{"温度测量值":sgl, "悬浮物测量值":sgl, "信号值":sgl})
          n127 = Unbundle By Name(w286) -> ("悬浮物测量值"=w285:sgl, "信号值"=w277:sgl)
          n128 = Unbundle By Name(w282) -> ("K"=w281:sgl, "B"=w280:sgl)
        }
      }
    }
    frame 3 {
      n129 = Unbundle By Name(w312) -> ("电导率探头选择"=w314:T1)
      n130 = case shown="\"STD\"" w314 {
        tunnel: [w318 w344 w379 w388] -> w313
        tunnel: [w324 w340 w378 w386] -> w311
        tunnel: w310 -> [w322 w348 _ _]
        tunnel: [w323 w349 w373 w385] -> w309
        tunnel: [w319 w345 w370 _] -> w308
        tunnel: [w316 w342 w369 _] -> w307
        tunnel: [_ _ _ TRUE] -> w306
        tunnel: [_ _ w368 w383] -> w304
        tunnel: [_ _ TRUE TRUE] -> w303
        tunnel: [_ _ w366 _] -> w302
        tunnel: ["%#.2f μS/cm" ("数值文本.格式字符串") "%#.2f μS/cm" ("数值文本.格式字符串") "%#.2f μS/cm" ("数值文本.格式字符串") "%#.6f" ("数值文本.格式字符串")] -> w301
        frame "禹山", Default {
          n131 = global read "多参数全局变量.vi" "重新获取KB值命令"() -> (w315:bool)
          n132 = case shown="False" w315 {
            tunnel: [w326 w330] -> w323
            tunnel: w322 -> [_ w335]
            tunnel: [w327 w329] -> w321
            tunnel: T3."电导率" ("探头") -> [_ w332]
            frame False {
              n133 = global read "多参数全局变量.vi" "禹山KB值"() -> (w328:T6)
              n134 = Unbundle By Name(w328) -> ("输出值"=w327:cluster{"K":sgl, "B":sgl}, "SN"=w326:string)
            }
            frame True {
              n135 = call "禹山获取用户校准参数.vi"("探头"=w332, "MB session in"=w335) -> ("error out"=w334:errorcluster, "输出值"=w329:cluster{"K":sgl, "B":sgl}, "MB session out"=w333:refnum<class "MB_Master.lvclass">)  [unwired: 7 in]
              n136 = call "禹山获取系列号.vi"("探头"=w332, "error in (no error)"=w334, "MB session in"=w333) -> ("error out"=w331:errorcluster, "SN"=w330:string)  [unwired: 6 in, 1 out]
              n137 = case shown="No Error" w331 {
                tunnel: w329 -> [w338 _]
                tunnel: w330 -> [w339 _]
                frame No Error {
                  n138 = Bundle("输出值"=w338, "SN"=w339) -> (w337:T6)  [unwired: 1 in]
                  n139 = global write "多参数全局变量.vi" "重新获取KB值命令"(FALSE ("重新获取KB值命令")) -> ()
                  n140 = global write "多参数全局变量.vi" "禹山KB值"(w337) -> ()
                }
                frame Error {
                }
              }
            }
          }
          n141 = global read "禹山过程全局变量.vi" "spcond"() -> (w325:cluster{"温度测量值":sgl, "测量值":sgl, "错误标志":u16})
          n142 = Unbundle By Name(w325) -> ("测量值"=w318:sgl)
          n143 = Unbundle By Name(w321) -> ("K"=w319:sgl, "B"=w316:sgl)
          n144 = formula code="Y=Y/1000;\nX = (Y-B)/K;\nX=X*1000;"("Y"=w318, "K"=w319, "B"=w316) -> ("X"=w324:dbl)
        }
        frame "STD" {
          n145 = global read "多参数全局变量.vi" "重新获取KB值命令"() -> (w341:bool)
          n146 = case shown="True" w341 {
            tunnel: [w351 w355] -> w349
            tunnel: w348 -> [_ w360]
            tunnel: [w352 w354] -> w347
            tunnel: T3."电导率" ("探头") -> [_ w357]
            frame False {
              n147 = global read "多参数全局变量.vi" "禹山KB值"() -> (w353:T6)
              n148 = Unbundle By Name(w353) -> ("输出值"=w352:cluster{"K":sgl, "B":sgl}, "SN"=w351:string)
            }
            frame True {
              n149 = call "STD获取用户校准参数.vi"("探头"=w357, "MB session in"=w360) -> ("error out"=w359:errorcluster, "输出值"=w354:cluster{"K":sgl, "B":sgl}, "MB session out"=w358:refnum<class "MB_Master.lvclass">)  [unwired: 7 in]
              n150 = call "STD获取系列号.vi"("探头"=w357, "error in (no error)"=w359, "MB session in"=w358) -> ("error out"=w356:errorcluster, "SN"=w355:string)  [unwired: 6 in, 1 out]
              n151 = case shown="No Error" w356 {
                tunnel: w354 -> [w363 _]
                tunnel: w355 -> [w364 _]
                frame No Error {
                  n152 = Bundle("输出值"=w363, "SN"=w364) -> (w362:T6)  [unwired: 1 in]
                  n153 = global write "多参数全局变量.vi" "重新获取KB值命令"(FALSE ("重新获取KB值命令")) -> ()
                  n154 = global write "多参数全局变量.vi" "禹山KB值"(w362) -> ()
                }
                frame Error {
                }
              }
            }
          }
          n155 = global read "禹山过程全局变量.vi" "STDspcond"() -> (w350:cluster{"温度测量值":sgl, "测量值":sgl, "信号值":sgl})
          n156 = Unbundle By Name(w350) -> ("测量值"=w344:sgl, "信号值"=w340:sgl)
          n157 = Unbundle By Name(w347) -> ("K"=w345:sgl, "B"=w342:sgl)
        }
        frame "国弘" {
          n158 = global read "国弘过程全局变量.vi" "Cond"() -> (w380:T13)
          n159 = Unbundle By Name(w380) -> ("电导率测量值"=w379:sgl, "电导率信号值"=w378:sgl, "生产批次"=w371:u16, "电极序号"=w372:u16, "电导率电极零点"=w369:sgl, "电导率电极斜率"=w370:sgl, "温度补偿系数"=w368:sgl, "电极状态标志"=w366:u16)
          n160 = Number To Decimal String(number=w371) -> (decimal integer string=w377:string)  [unwired: 1 in]
          n161 = Number To Decimal String(number=w372) -> (decimal integer string=w375:string)  [unwired: 1 in]
          n162 = Concatenate Strings("MQ" ("字符串"), w377, "02" ("字符串"), w375) -> (w373:string)
        }
        frame "纳清" {
          n163 = global read "纳清过程全局变量.vi" "电导率测试值"() -> (w387:T14)
          n164 = Unbundle By Name(w387) -> ("电导率数据（uS/cm）"=w388:sgl, "电导率原始信号电阻"=w386:sgl, "序列号"=w385:string, "温度补偿系数"=w383:sgl)
        }
      }
    }
    frame 4 {
      n165 = Unbundle By Name(w397) -> ("叶绿素a探头选择"=w399:T1)
      n166 = case shown="\"禹山\", Default" w399 {
        tunnel: [w409 w434 w453 w459] -> w398
        tunnel: [w408 w425 w453 w457] -> w396
        tunnel: w395 -> [w406 w432 _ _]
        tunnel: [w407 w433 "" ("序列号") w456] -> w394
        tunnel: [w403 w429 _ _] -> w393
        tunnel: [w402 w428 _ _] -> w392
        tunnel: [_ _ TRUE TRUE] -> w391
        tunnel: ["%#.2f μg/L" ("数值文本.格式字符串") "%#.2f μg/L" ("数值文本.格式字符串") "%#.2f μg/L" ("数值文本.格式字符串") "%#.6f" ("数值文本.格式字符串")] -> w389
        frame "禹山", Default {
          n167 = global read "多参数全局变量.vi" "重新获取KB值命令"() -> (w400:bool)
          n168 = case shown="True" w400 {
            tunnel: [w411 w414] -> w407
            tunnel: w406 -> [_ w420]
            tunnel: [w412 w415] -> w405
            tunnel: T3."叶绿素a" ("探头") -> [_ w417]
            frame False {
              n169 = global read "多参数全局变量.vi" "禹山KB值"() -> (w413:T6)
              n170 = Unbundle By Name(w413) -> ("输出值"=w412:cluster{"K":sgl, "B":sgl}, "SN"=w411:string)
            }
            frame True {
              n171 = call "禹山获取用户校准参数.vi"("探头"=w417, "MB session in"=w420) -> ("error out"=w418:errorcluster, "输出值"=w415:cluster{"K":sgl, "B":sgl}, "MB session out"=w419:refnum<class "MB_Master.lvclass">)  [unwired: 7 in]
              n172 = call "禹山获取系列号.vi"("探头"=w417, "error in (no error)"=w418, "MB session in"=w419) -> ("error out"=w416:errorcluster, "SN"=w414:string)  [unwired: 6 in, 1 out]
              n173 = case shown="No Error" w416 {
                tunnel: w415 -> [w424 _]
                tunnel: w414 -> [w421 _]
                frame No Error {
                  n174 = Bundle("输出值"=w424, "SN"=w421) -> (w423:T6)  [unwired: 1 in]
                  n175 = global write "多参数全局变量.vi" "重新获取KB值命令"(FALSE ("重新获取KB值命令")) -> ()
                  n176 = global write "多参数全局变量.vi" "禹山KB值"(w423) -> ()
                }
                frame Error {
                }
              }
            }
          }
          n177 = global read "禹山过程全局变量.vi" "叶绿素a"() -> (w410:cluster{"温度测量值":sgl, "叶绿素测量值":sgl, "错误标志":u16})
          n178 = Unbundle By Name(w410) -> ("叶绿素测量值"=w409:sgl)
          n179 = Unbundle By Name(w405) -> ("K"=w403:sgl, "B"=w402:sgl)
          n180 = formula code="X = (Y-B)/K;"("Y"=w409, "K"=w403, "B"=w402) -> ("X"=w408:dbl)
        }
        frame "STD" {
          n181 = global read "多参数全局变量.vi" "重新获取KB值命令"() -> (w426:bool)
          n182 = case shown="True" w426 {
            tunnel: [w436 w439] -> w433
            tunnel: w432 -> [_ w445]
            tunnel: [w437 w440] -> w431
            tunnel: T3."叶绿素a" ("探头") -> [_ w442]
            frame False {
              n183 = global read "多参数全局变量.vi" "禹山KB值"() -> (w438:T6)
              n184 = Unbundle By Name(w438) -> ("输出值"=w437:cluster{"K":sgl, "B":sgl}, "SN"=w436:string)
            }
            frame True {
              n185 = call "STD获取用户校准参数.vi"("探头"=w442, "MB session in"=w445) -> ("error out"=w443:errorcluster, "输出值"=w440:cluster{"K":sgl, "B":sgl}, "MB session out"=w444:refnum<class "MB_Master.lvclass">)  [unwired: 7 in]
              n186 = call "STD获取系列号.vi"("探头"=w442, "error in (no error)"=w443, "MB session in"=w444) -> ("error out"=w441:errorcluster, "SN"=w439:string)  [unwired: 6 in, 1 out]
              n187 = case shown="No Error" w441 {
                tunnel: w440 -> [w449 _]
                tunnel: w439 -> [w446 _]
                frame No Error {
                  n188 = Bundle("输出值"=w449, "SN"=w446) -> (w448:T6)  [unwired: 1 in]
                  n189 = global write "多参数全局变量.vi" "重新获取KB值命令"(FALSE ("重新获取KB值命令")) -> ()
                  n190 = global write "多参数全局变量.vi" "禹山KB值"(w448) -> ()
                }
                frame Error {
                }
              }
            }
          }
          n191 = global read "禹山过程全局变量.vi" "STD叶绿素a"() -> (w435:cluster{"温度测量值":sgl, "叶绿素测量值":sgl, "信号值":sgl})
          n192 = Unbundle By Name(w435) -> ("叶绿素测量值"=w434:sgl, "信号值"=w425:sgl)
          n193 = Unbundle By Name(w431) -> ("K"=w429:sgl, "B"=w428:sgl)
        }
        frame "国弘" {
          w453 = sgl 0.0 ("温度数据")
        }
        frame "纳清" {
          n194 = global read "纳清过程全局变量.vi" "叶绿素a测试值"() -> (w458:T15)
          n195 = Unbundle By Name(w458) -> ("叶绿素a"=w459:sgl, "原始光强数值"=w457:u16, "序列号"=w456:string)
        }
      }
    }
    frame 5 {
      n196 = Unbundle By Name(w468) -> ("蓝绿藻探头选择"=w470:T1)
      n197 = case shown="\"STD\"" w470 {
        tunnel: [w474 w479 w504 w510] -> w469
        tunnel: [w474 w478 w504 w508] -> w467
        tunnel: ["" ("序列号") w475 "" ("序列号") w507] -> w466
        tunnel: [TRUE FALSE TRUE TRUE] -> w465
        tunnel: ["%#.2f cells/mL" ("数值文本.格式字符串") "%#.2f cells/mL" ("数值文本.格式字符串") "%#.2f cells/mL" ("数值文本.格式字符串") "%#.6f" ("数值文本.格式字符串")] -> w463
        tunnel: w462 -> [_ w480 _ _]
        tunnel: [_ w477 _ _] -> w461
        tunnel: [_ w476 _ _] -> w460
        frame "禹山", Default {
          w474 = sgl 0.0 ("温度数据")
        }
        frame "STD" {
          n198 = global read "多参数全局变量.vi" "重新获取KB值命令"() -> (w484:bool)
          n199 = case shown="True" w484 {
            tunnel: [w487 w490] -> w475
            tunnel: w480 -> [_ w496]
            tunnel: [w488 w491] -> w483
            tunnel: T5."藻密度" ("探头") -> [_ w493]
            frame False {
              n200 = global read "多参数全局变量.vi" "禹山KB值"() -> (w489:T6)
              n201 = Unbundle By Name(w489) -> ("输出值"=w488:cluster{"K":sgl, "B":sgl}, "SN"=w487:string)
            }
            frame True {
              n202 = call "STD获取用户校准参数.vi"("探头"=w493, "MB session in"=w496) -> ("error out"=w494:errorcluster, "输出值"=w491:cluster{"K":sgl, "B":sgl}, "MB session out"=w495:refnum<class "MB_Master.lvclass">)  [unwired: 7 in]
              n203 = call "STD获取系列号.vi"("探头"=w493, "error in (no error)"=w494, "MB session in"=w495) -> ("error out"=w492:errorcluster, "SN"=w490:string)  [unwired: 6 in, 1 out]
              n204 = case shown="No Error" w492 {
                tunnel: w491 -> [w500 _]
                tunnel: w490 -> [w497 _]
                frame No Error {
                  n205 = Bundle("输出值"=w500, "SN"=w497) -> (w499:T6)  [unwired: 1 in]
                  n206 = global write "多参数全局变量.vi" "重新获取KB值命令"(FALSE ("重新获取KB值命令")) -> ()
                  n207 = global write "多参数全局变量.vi" "禹山KB值"(w499) -> ()
                }
                frame Error {
                }
              }
            }
          }
          n208 = global read "禹山过程全局变量.vi" "STD藻密度"() -> (w482:cluster{"温度测量值":sgl, "测量值":sgl, "信号值":sgl})
          n209 = Unbundle By Name(w482) -> ("测量值"=w479:sgl, "信号值"=w478:sgl)
          n210 = Unbundle By Name(w483) -> ("K"=w477:sgl, "B"=w476:sgl)
        }
        frame "国弘" {
          w504 = sgl 0.0 ("温度数据")
        }
        frame "纳清" {
          n211 = global read "纳清过程全局变量.vi" "蓝绿藻测试值"() -> (w509:T16)
          n212 = Unbundle By Name(w509) -> ("蓝绿藻"=w510:sgl, "原始光强数值"=w508:u16, "序列号"=w507:string)
        }
      }
    }
    frame 6 {
      n213 = Unbundle By Name(w519) -> ("orp探头选择"=w521:T1)
      n214 = case shown="\"禹山\", Default" w521 {
        tunnel: [w524 w535 w539] -> w520
        tunnel: [w524 w534 w539] -> w518
        tunnel: ["" w527 ""] -> w517
        tunnel: [TRUE TRUE TRUE] -> w516
        tunnel: [_ w525 _] -> w512
        frame "禹山", Default {
          w524 = sgl 0.0 ("温度数据")
        }
        frame "国弘" {
          n215 = global read "国弘过程全局变量.vi" "ORP"() -> (w536:T17)
          n216 = Unbundle By Name(w536) -> ("测量值"=w535:sgl, "信号值"=w534:sgl, "生产批次"=w528:u16, "传感器序号"=w529:u16, "电极状态标志"=w525:u16)
          n217 = Number To Decimal String(number=w528) -> (decimal integer string=w533:string)  [unwired: 1 in]
          n218 = Number To Decimal String(number=w529) -> (decimal integer string=w531:string)  [unwired: 1 in]
          n219 = Concatenate Strings("MQ" ("字符串"), w533, "05" ("字符串"), w531) -> (w527:string)
        }
        frame "纳清" {
          w539 = sgl 0.0 ("温度测量值")
        }
      }
    }
    frame 7 {
      n220 = global read "国弘过程全局变量.vi" "COD"() -> (w546:T18)
      n221 = Unbundle By Name(w546) -> ("电极状态标志"=w548:u16, "COD测量值"=w554:sgl, "COD信号值"=w553:sgl, "生产批次"=w541:u16, "电极序号"=w540:u16, "COD零点系数"=w550:sgl, "COD斜率系数"=w551:sgl)
      n222 = Number To Decimal String(number=w541) -> (decimal integer string=w545:string)  [unwired: 1 in]
      n223 = Number To Decimal String(number=w540) -> (decimal integer string=w543:string)  [unwired: 1 in]
      n224 = Concatenate Strings("MQ" ("字符串"), w545, "08" ("字符串"), w543) -> (w552:string)
    }
    frame 8 {
      n225 = global read "多参数全局变量.vi" "重新获取KB值命令"() -> (w555:bool)
      n226 = case shown="False" w555 {
        tunnel: [w569 w571] -> w564
        tunnel: w563 -> [_ w577]
        tunnel: [w568 w572] -> w562
        tunnel: T3."DO2" ("探头") -> [_ w574]
        frame False {
          n227 = global read "多参数全局变量.vi" "禹山KB值"() -> (w570:T6)
          n228 = Unbundle By Name(w570) -> ("输出值"=w568:cluster{"K":sgl, "B":sgl}, "SN"=w569:string)
        }
        frame True {
          n229 = call "禹山获取用户校准参数.vi"("探头"=w574, "MB session in"=w577) -> ("error out"=w576:errorcluster, "输出值"=w572:cluster{"K":sgl, "B":sgl}, "MB session out"=w575:refnum<class "MB_Master.lvclass">)  [unwired: 7 in]
          n230 = call "禹山获取系列号.vi"("探头"=w574, "error in (no error)"=w576, "MB session in"=w575) -> ("error out"=w573:errorcluster, "SN"=w571:string)  [unwired: 6 in, 1 out]
          n231 = case shown="No Error" w573 {
            tunnel: w572 -> [w580 _]
            tunnel: w571 -> [w581 _]
            frame No Error {
              n232 = Bundle("输出值"=w580, "SN"=w581) -> (w579:T6)  [unwired: 1 in]
              n233 = global write "多参数全局变量.vi" "重新获取KB值命令"(FALSE ("重新获取KB值命令")) -> ()
              n234 = global write "多参数全局变量.vi" "禹山KB值"(w579) -> ()
            }
            frame Error {
            }
          }
        }
      }
      n235 = global read "禹山过程全局变量.vi" "DO 2"() -> (w567:cluster{"温度测量值":sgl, "DO%":sgl, "DOmg/L":sgl})
      n236 = Unbundle By Name(w567) -> ("DO%"=w565:sgl)
      n237 = Unbundle By Name(w562) -> ("K"=w559:sgl, "B"=w558:sgl)
      n238 = formula code="Y = Y / 100;\nX = (Y-B)/K;\nX = 100 * X;"("Y"=w565, "K"=w559, "B"=w558) -> ("X"=w566:dbl)
    }
    frame 9 {
      n239 = global read "国弘过程全局变量.vi" "氯化物"() -> (w588:T19)
      n240 = Unbundle By Name(w588) -> ("电极状态标志"=w590:u16, "测量值"=w596:sgl, "信号值"=w595:sgl, "生产批次"=w583:u16, "电极序号"=w582:u16, "电极零点"=w592:sgl, "电极斜率"=w593:sgl)
      n241 = Number To Decimal String(number=w583) -> (decimal integer string=w587:string)  [unwired: 1 in]
      n242 = Number To Decimal String(number=w582) -> (decimal integer string=w585:string)  [unwired: 1 in]
      n243 = Concatenate Strings("MQ" ("字符串"), w587, "01" ("字符串"), w585) -> (w594:string)
    }
    frame 10 {
      n244 = global read "纳清过程全局变量.vi" "氨氮测试值"() -> (w597:T20)
      n245 = Unbundle By Name(w597) -> ("参数2数据"=w603:sgl, "参数2原始信号"=w602:sgl, "序列号"=w601:string)
    }
    frame 11 {
      n246 = global read "国弘过程全局变量.vi" "水中油"() -> (w610:T21)
      n247 = Unbundle By Name(w610) -> ("电极状态标志"=w612:u16, "测量值"=w618:sgl, "信号值"=w617:sgl, "生产批次"=w605:u16, "电极序号"=w604:u16, "水中油零点系数"=w614:sgl, "水中油斜率系数"=w615:sgl)
      n248 = Number To Decimal String(number=w605) -> (decimal integer string=w609:string)  [unwired: 1 in]
      n249 = Number To Decimal String(number=w604) -> (decimal integer string=w607:string)  [unwired: 1 in]
      n250 = Concatenate Strings("MQ" ("字符串"), w609, "17" ("字符串"), w607) -> (w616:string)
    }
  }
  "检测值" <- w17
  "信号值" <- w14
  "序列号" <- w12
  "检测值.格式字符串" <- w6
  "电极状态标志" <- w2
  "信号值.格式字符串" <- w1
  n251 = Not(x=w11) -> (.not. x?=w10:bool)
  n252 = Bundle(w5, "温度补偿系数"=w4) -> (→"温度补偿系数":cluster{bool, "温度补偿系数":sgl})  [unwired: 1 in]
  n253 = Bundle(w10, "水中油斜率系数"=w9, "水中油零点系数"=w8) -> (→"线性系数":cluster{bool, "水中油斜率系数":sgl, "水中油零点系数":sgl})  [unwired: 1 in]
